vi "Set Intake Cmd.vi"(8 "error in":errorcluster, 11 "Cmd":T1) -> (0 "error out":errorcluster)   [LabVIEW 2016, in "Intake.lvlib"]
uses:
  Intake.lvlib
  Typedef/Intake Command.ctl
  Typedef/Intake Msg.ctl
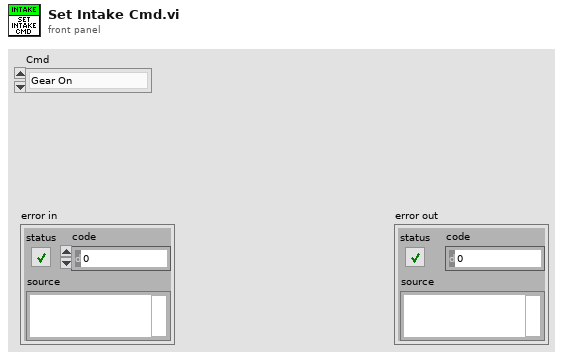
[diagram p1: front panel]
types:
  T1 = typedef "Intake.lvlib/Intake Command.ctl" = enum16{"Gear On", "Gear Off", "Gear Reverse", "Gear Retract", "Gear Deploy", "All Off", "All Off Closed", "Fuel Deploy", "Fuel Retract", "Fuel Agitate", "Fuel Reverse"}
  T2 = typedef "Intake.lvlib/Intake Msg.ctl" = cluster{"Cmd":T1, "Variant":variant}
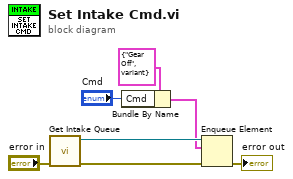
[diagram p0: block diagram]
diagram:
  n1 = call "Get Intake Queue.vi"("error in"="error in") -> ("error out"=w5:errorcluster, "queue out"=w7:refnum<queue>)  [unwired: 9 in]
  n2 = Bundle By Name(cluster=T2 {"Cmd"=enum."Gear Off", "Variant"=variant} ("element"), "Cmd"="Cmd") -> (w2:T2)
  n3 = Enqueue Element(queue=w7, element=w2, error in (no error)=w5) -> (error out=→"error out":errorcluster)  [unwired: 1 in, 2 out]
